vi "Write Tooltip.vi"(8 "error in (no error)":errorcluster, 10 "Tooltip":string, 11 "GridColumn in":refnum<class "GridColumn.lvclass">) -> (0 "error out":errorcluster, 3 "GridColumn out":refnum<class "GridColumn.lvclass">)   [LabVIEW 2016, in "DataGrid.lvlib" / "GridColumn.lvclass"]
uses:
  <userlib>/LabVIEWdotNetDataGrid/source/GridColumn/GridColumn.lvclass
  <userlib>/LabVIEWdotNetDataGrid/source/GridColumn/GridColumn.lvclass/GridColumn.ctl
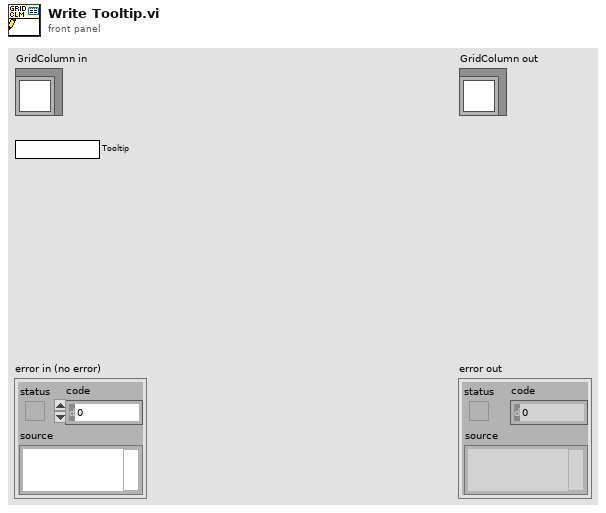
[diagram p1: front panel]
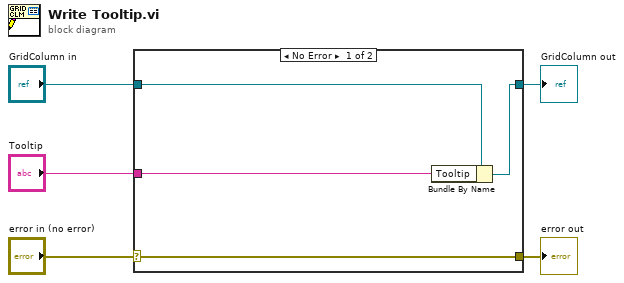
[diagram p0: block diagram]
diagram:
  n1 = case shown="No Error" "error in (no error)" {
    selector: "error in (no error)" -> [w9 w10]
    tunnel: [w9 w10] -> w4
    tunnel: [w7 w11] -> w2
    tunnel: "GridColumn in" -> [w8 w11]
    tunnel: "Tooltip" -> [w6 _]
    frame No Error {
      n2 = Bundle By Name(cluster=w8, "Tooltip"=w6) -> (w7:refnum<class "GridColumn.lvclass">)
    }
    frame Error {
    }
  }
  "error out" <- w4
  "GridColumn out" <- w2
